vi "test Read Properties.vi"(8 "error in (no error)":errorcluster, 11 "TestCase in":refnum<class "SLSC EDS System Tests.lvclass">) -> (0 "error out":errorcluster, 3 "TestCase out":refnum<class "SLSC EDS System Tests.lvclass">)   [LabVIEW 2015, in "SLSC EDS System Tests.lvclass"]
uses:
  SLSC EDS System Tests.lvclass
  SLSC EDS API/JSON parsing/EDSjsonStructure.ctl
  SLSC EDS API/JSON parsing/enum.ctl
  SLSC EDS API/JSON parsing/property.ctl
  SLSC EDS API/JSON parsing/command.ctl
  SLSC EDS API/JSON parsing/scale.ctl
  SLSC EDS API/JSON parsing/physicalChannel.ctl
  SLSC EDS API/JSON parsing/register.ctl
  SLSC EDS System Tests.lvclass/SLSC EDS System Tests.ctl
  <vilib>/addons/_JKI Toolkits/VI Tester/TestCase.llb/TestCase.lvclass
  SLSC EDS API/SLSC EDS API.lvlib
panel:
  out "SLSC EDS module out":T1
  # "not working\nregisterMap->registers->initialValue"
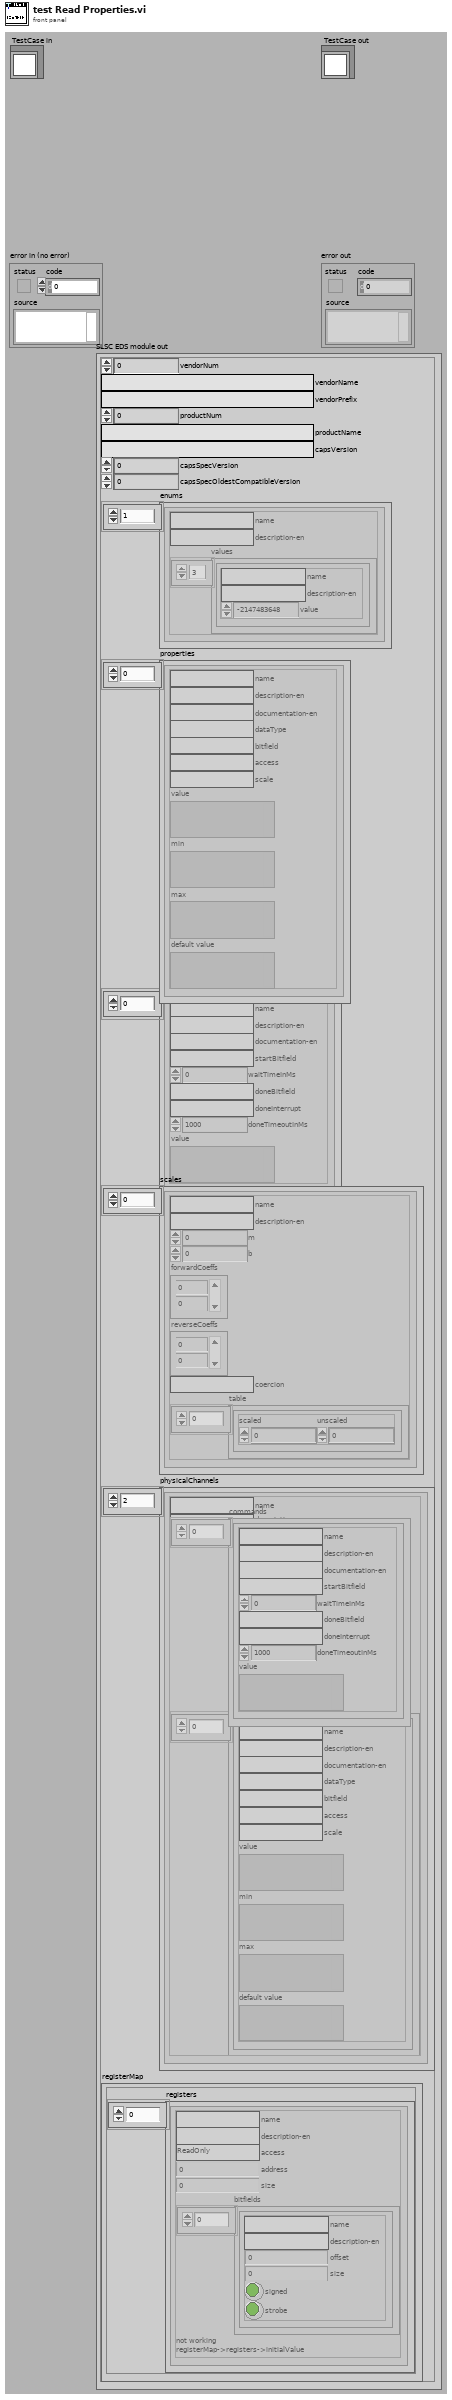
[diagram p1: front panel]
types:
  T1 = typedef "EDSjsonStructure.ctl" = cluster{"vendorNum":u32, "vendorName":string, "vendorPrefix":string, "productNum":u32, "productName":string, "capsVersion":string, "capsSpecVersion":u32, "capsSpecOldestCompatibleVersion":u32, "enums":T2[], "properties":T3[], "commands":T4[], "scales":T5[], "physicalChannels":T6[], "registerMap":cluster{"registers":T7[]}}
  T2 = typedef "enum.ctl" = cluster{"name":string, "description-en":string, "values":cluster{"name":string, "description-en":string, "value":i32}[]}
  T3 = typedef "property.ctl" = cluster{"name":string, "description-en":string, "documentation-en":string, "dataType":string, "bitfield":string, "access":string, "scale":string, "value":variant, "min":variant, "max":variant, "default value":variant}
  T4 = typedef "command.ctl" = cluster{"name":string, "description-en":string, "documentation-en":string, "startBitfield":string, "waitTimeInMs":i32, "doneBitfield":string, "doneInterrupt":string, "doneTimeoutInMs":i32, "value":variant}
  T5 = typedef "scale.ctl" = cluster{"name":string, "description-en":string, "m":dbl, "b":dbl, "forwardCoeffs":dbl[], "reverseCoeffs":dbl[], "coercion":string, "table":cluster{"scaled":dbl, "unscaled":dbl}[]}
  T6 = typedef "physicalChannel.ctl" = cluster{"name":string, "description-en":string, "commands":T4[], "properties":T3[]}
  T7 = typedef "register.ctl" = cluster{"name":string, "description-en":string, "access":string, "address":u32, "size":u32, "bitfields":cluster{"name":string, "description-en":string, "offset":u32, "size":u32, "signed":bool, "strobe":bool}[]}
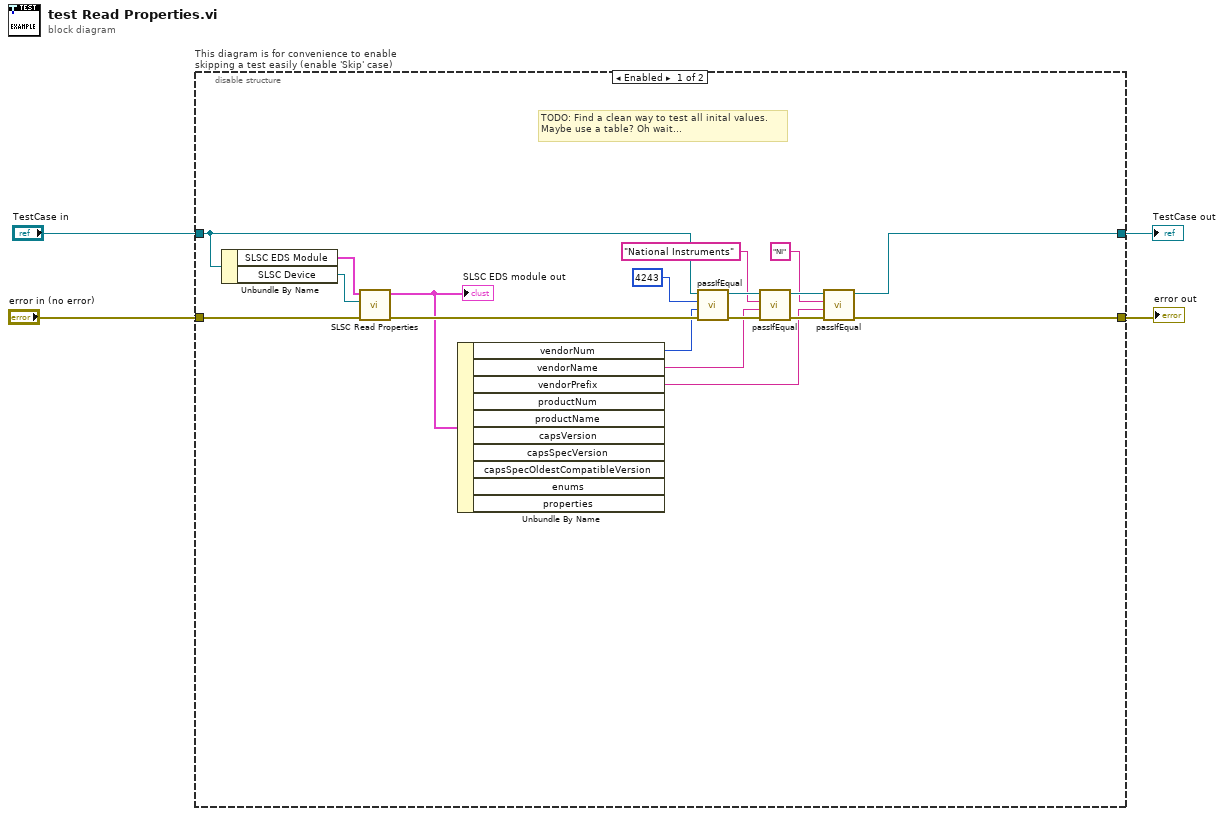
[diagram p0: block diagram]
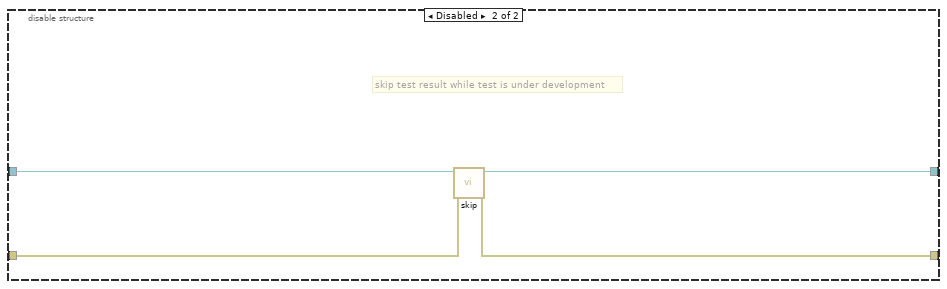
[diagram p2: hidden frame]
diagram:
  n1 = disable-structure "This diagram is for convenience to enable skipping a test easily (enable 'Skip' case)" shown="Enabled" {
    disable-tunnel: "TestCase in" -> [w17 w25]
    disable-tunnel: [w7 w23] -> w1
    disable-tunnel: [w8 w24] -> w3
    disable-tunnel: "error in (no error)" -> [w19 w22]
    frame Enabled {
      # "TODO: Find a clean way to test all inital values.\nMaybe use a table? Oh wait..."
      n2 = Unbundle By Name(w17) -> ("SLSC EDS Module"=w21:T1, "SLSC Device"=w20:refnum<k21>)
      n3 = call "SLSC Read Properties.vi"("error in (no error)"=w19, "SLSC Device"=w20, "SLSC EDS module in"=w21) -> ("error out"=w18:errorcluster, "SLSC EDS module out"=w16:T1)  [unwired: 7 in]
      "SLSC EDS module out" <- w16
      n4 = Unbundle By Name(w16) -> ("vendorNum"=w12:u32, "vendorName"=w10:string, "vendorPrefix"=w6:string)  [unwired: 7 out]
      n5 = call-dynamic "passIfEqual.vi"("error in (no error)"=w18, "y"=w12, "x"=u32 4243, "TestCase in"=w17) -> ("error out"=w11:errorcluster, "TestCase out"=w15:refnum<class "SLSC EDS System Tests.lvclass">)  [unwired: 6 in]
      n6 = call-dynamic "passIfEqual.vi"("error in (no error)"=w11, "y"=w10, "x"="National Instruments", "TestCase in"=w15) -> ("error out"=w8:errorcluster, "TestCase out"=w14:refnum<class "SLSC EDS System Tests.lvclass">)  [unwired: 6 in]
      n7 = call-dynamic "passIfEqual.vi"("y"=w6, "x"="NI", "TestCase in"=w14) -> ("TestCase out"=w7:refnum<class "SLSC EDS System Tests.lvclass">)  [unwired: 7 in, 1 out]
    }
    frame Disabled {
      # "skip test result while test is under development"
      n8 = call <vilib>:"skip.vi"("error in (no error)"=w22, "TestCase in"=w25) -> ("error out"=w24:errorcluster, "TestCase out"=w23:refnum<class "SLSC EDS System Tests.lvclass">)  [unwired: 8 in]
    }
  }
  "error out" <- w3
  "TestCase out" <- w1
